vi "Encode File as Base64.vi"(8 "error in":errorcluster, 10 "file":path) -> (0 "error out":errorcluster, 2 "string out (base64-encoded)":string)   [LabVIEW 2013]
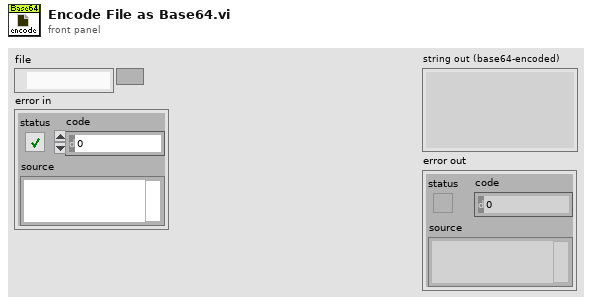
[diagram p1: front panel]
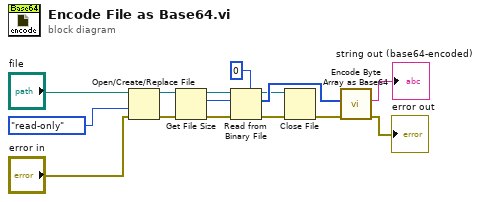
[diagram p0: block diagram]
diagram:
  n1 = Open/Create/Replace File(file path (use dialog)="file", error in="error in", access (0:read/write)=enum16{"read/write", "read-only", "write-only"}."read-only") -> (refnum out=w9:refnum<file>, error out=w10:errorcluster)  [unwired: 3 in, 1 out]
  n2 = Get File Size(file=w9, error in=w10) -> (refnum out=w15:refnum<file>, size (in bytes)=w13:i64, 0:w14:errorcluster)
  n3 = Read from Binary File(5:u8 0, 8:w14, 10:w13, 11:w15) -> (0:w5:errorcluster, 2:w11:u8[], 3:w4:refnum<file>)  [unwired: 2 in, 1 out]
  n4 = Close File(refnum=w4, error in=w5) -> (error out=w2:errorcluster)  [unwired: 1 out]
  n5 = call "Encode Byte Array as Base64.vi"("error in (no error)"=w2, "unsigned byte array"=w11) -> ("error out"=→"error out":errorcluster, "string out (base64-encoded)"=→"string out (base64-encoded)":string)  [unwired: 8 in]
